vi "global-CSMQ FGV Change Flag.vi"() -> ()   [LabVIEW 2020, in "Communicable State Machine.lvlib"]
uses:
  Communicable State Machine.lvlib
panel:
  in  "global-CSMQ FGV Change Flag":u64=4603270806574966694 format="%08x"
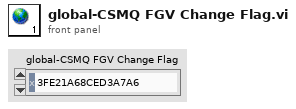
[diagram p1: front panel]
diagram:
